vi "Über.vi"(11 "version":string) -> ()   [LabVIEW 2010]
panel:
  out "String":string
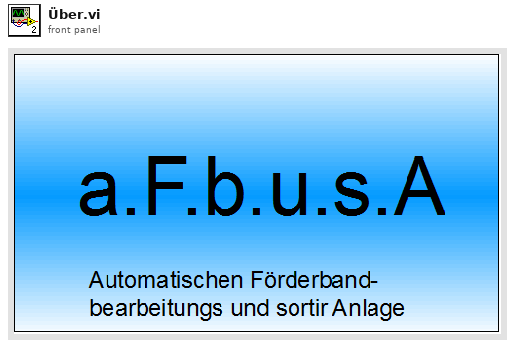
[diagram p1: front panel]
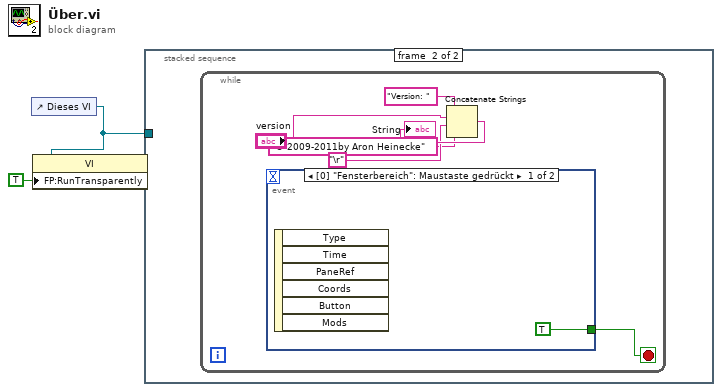
[diagram p0: block diagram]
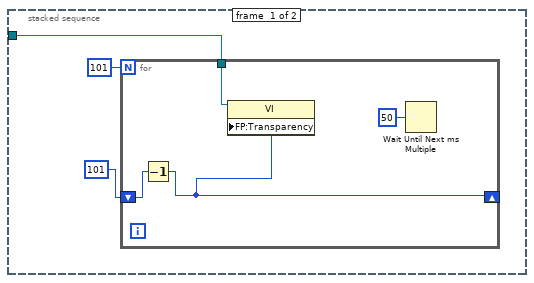
[diagram p2: hidden frame]
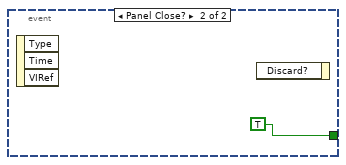
[diagram p3: hidden frame]
diagram:
  n1 = control-ref of="Dieses VI"() -> (w2:refnum<vi>)
  n2 = property class="VI"(reference=w2, "FP:RunTransparently"=TRUE ("Frontpanel-Fenster:VI transparent ausführen")) -> ()  [unwired: 1 in, 2 out]
  n3 = stacked-sequence {
    tunnel: w2 -> [w3 _]
    frame #0 {
      n4 = for {
        N: 101 -> [_]
        shift-right: [w8] -> _
        shift-left: 101 -> [w9]
        tunnel: w3 -> [w6]
        n5 = Decrement(x=w9) -> (x-1=w8:i32)
        n6 = property class="VI"(reference=w6, "FP:Transparency"=w8) -> ()  [unwired: 1 in, 2 out]
        n7 = Wait Until Next ms Multiple(millisecond multiple=u32 50 ("Vielfache von ms")) -> ()  [unwired: 1 out]
      }
    }
    frame #1 {
      n8 = while {
        stop <- w12 stop-if-true
        n9 = event shown="[0] \"Fensterbereich\": Maustaste gedrückt" {
          selector: _ -> [_ _]
          dyn-events: _ -> [_ _]
          timeout: _ -> [_ _]
          tunnel: [TRUE TRUE] -> w12
          event Mouse Down {
            n10 = event-data() -> ()  [unwired: 7 out]
          }
          event Panel Close? {
            n11 = event-data() -> ()  [unwired: 4 out]
            n12 = event-data() -> ()  [unwired: 2 in, 1 out]
          }
        }
        n13 = Concatenate Strings("Version: " ("String"), "version", "\r", "© 2009-2011by Aron Heinecke" ("String")) -> (→"String":string)
      }
    }
  }
